vi "All Unit Tests.vi"(8 "error in (no error)":errorcluster) -> (0 "error out":errorcluster)   [LabVIEW 2026, in "Tests.lvlib"]
doc: "Aggregator for the Lumberjack unit tier. Holds every pure-VI unit test as a parallel subVI so the whole tier runs from one call. Has no assertions itself; each child registers its own via Define Test. Run directly for a fast, fixture-free unit-only pass (interactive Caraya dialog), or let Test.vi call it inside the suite for a headless, reported run. Add a unit test by dropping it here in parallel (Test-Strategy 3.2, 6)."
uses:
  Tests.lvlib
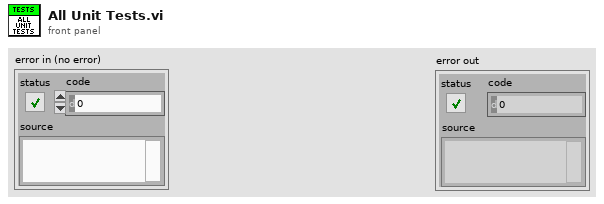
[diagram p1: front panel]
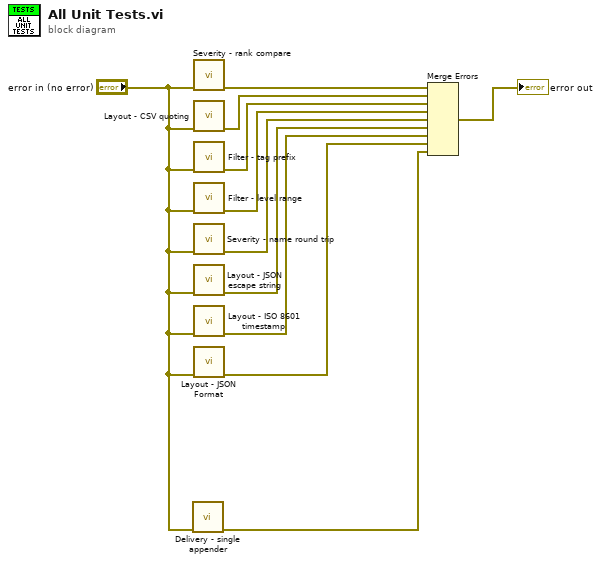
[diagram p0: block diagram]
diagram:
  n1 = call "Delivery - single appender.vi"("error in (no error)"="error in (no error)") -> ("error out"=w1:errorcluster)  [unwired: 10 in]
  n2 = call "Severity - rank compare.vi"("error in (no error)"="error in (no error)") -> ("error out"=w11:errorcluster)  [unwired: 10 in]
  n3 = call "Layout - CSV quoting.vi"("error in (no error)"="error in (no error)") -> ("error out"=w9:errorcluster)  [unwired: 10 in]
  n4 = call "Filter - tag prefix.vi"("error in (no error)"="error in (no error)") -> ("error out"=w8:errorcluster)  [unwired: 10 in]
  n5 = call "Filter - level range.vi"("error in (no error)"="error in (no error)") -> ("error out"=w7:errorcluster)  [unwired: 10 in]
  n6 = call "Severity - name round trip.vi"("error in (no error)"="error in (no error)") -> ("error out"=w6:errorcluster)  [unwired: 10 in]
  n7 = call "Layout - JSON escape string.vi"("error in (no error)"="error in (no error)") -> ("error out"=w5:errorcluster)  [unwired: 10 in]
  n8 = call "Layout - ISO 8601 timestamp.vi"("error in (no error)"="error in (no error)") -> ("error out"=w4:errorcluster)  [unwired: 10 in]
  n9 = call "Layout - JSON Format.vi"("error in (no error)"="error in (no error)") -> ("error out"=w3:errorcluster)  [unwired: 10 in]
  n10 = Merge Errors(w11, w9, w8, w7, w6, w5, w4, w3, w1) -> (→"error out":errorcluster)
